vi "ButtonPress.vi"(1 "Input":bool) -> (0 "Output":bool)   [LabVIEW 2019]
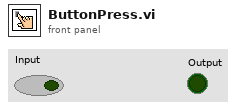
[diagram p1: front panel]
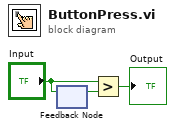
[diagram p0: block diagram]
diagram:
  n1 = feedback-in #1("Input") -> ()
  n2 = feedback #1() -> (w1:bool)  [unwired: 1 in]
  n3 = Greater?(x="Input", y=w1) -> (0:→"Output":bool)
